vi "HEWH RLT Error Checker.vi"(0 "A Data Array":string[][](array[string]), 1 "Disable Station 1":T1, 2 "Disable Station 2":T1, 5 "B Data Array":string[][](array[string]), 7 "C Data Array":string[][](array[string]), 9 "D Data Array":string[][](array[string]), 11 "Error In":errorcluster, 12 "Disable Station 3":T1, 13 "Disable Station 4":T1) -> (4 "Alarm A":bool, 6 "Alarm B":bool, 8 "Alarm C":bool, 10 "Alarm D":bool, 15 "Error Out":errorcluster)   [LabVIEW 2016]
uses:
  Type Definitions/HEWH RLT Station Disable.ctl
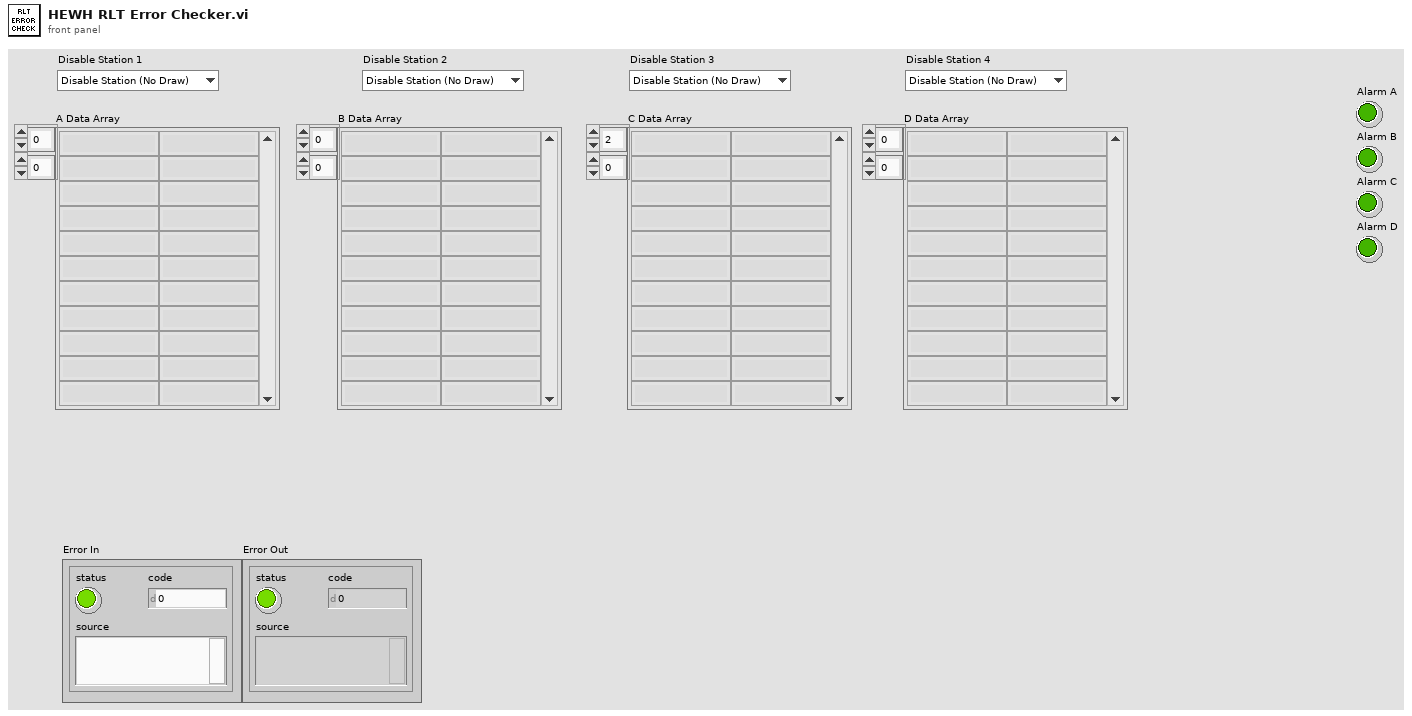
[diagram p1: front panel]
types:
  T1 = typedef "HEWH RLT Station Disable.ctl" = enum16{"Disable Station (No Draw)", "Enable Station"}
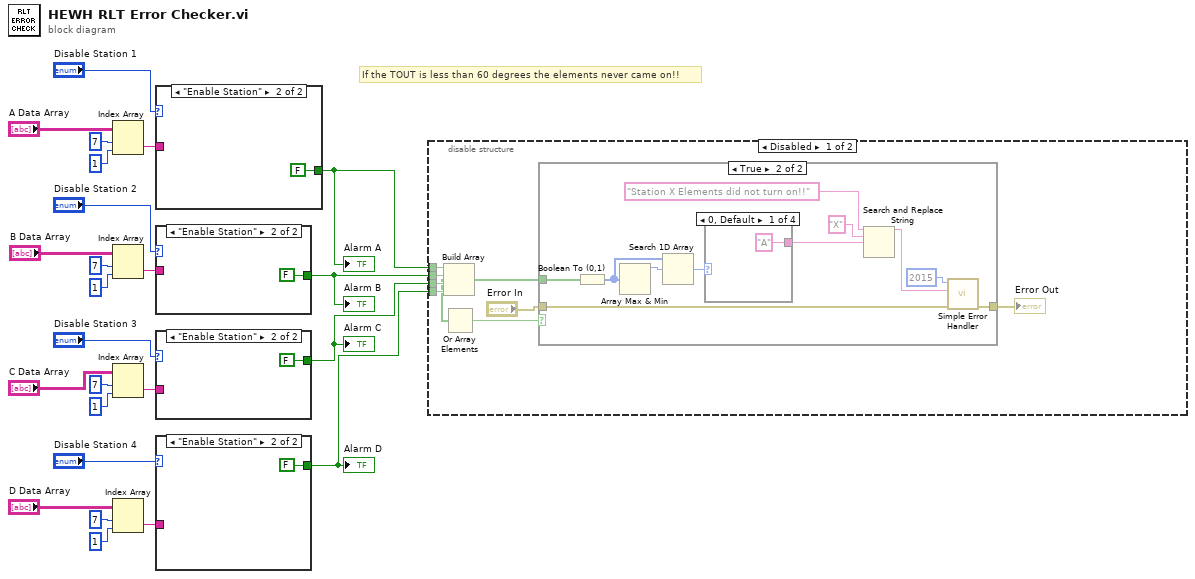
[diagram p0: block diagram]
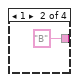
[diagram p3: hidden frame]
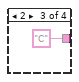
[diagram p4: hidden frame]
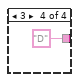
[diagram p5: hidden frame]
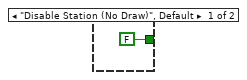
[diagram p7: hidden frame]
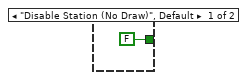
[diagram p8: hidden frame]
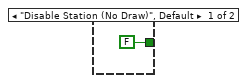
[diagram p9: hidden frame]
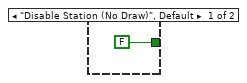
[diagram p10: hidden frame]
diagram:
  # "If the TOUT is less than 60 degrees the elements never came on!!"
  n1 = Index Array(array="A Data Array", index (row)=7 ("disabled index (row)"), index (col)=1 ("disabled index (col)")) -> (element=w11:string)
  n2 = Index Array(array="B Data Array", index (row)=7 ("disabled index (row)"), index (col)=1 ("disabled index (col)")) -> (element=w8:string)
  n3 = Index Array(array="C Data Array", index (row)=7 ("disabled index (row)"), index (col)=1 ("disabled index (col)")) -> (element=w9:string)
  n4 = Index Array(array="D Data Array", index (row)=7 ("disabled index (row)"), index (col)=1 ("disabled index (col)")) -> (element=w10:string)
  n5 = case shown="\"Enable Station\"" "Disable Station 1" {
    tunnel: w11 -> [_ _]
    tunnel: [FALSE FALSE] -> w4
    frame "Disable Station (No Draw)", Default {
    }
    frame "Enable Station" {
    }
  }
  "Alarm A" <- w4
  n6 = case shown="\"Enable Station\"" "Disable Station 2" {
    tunnel: w8 -> [_ _]
    tunnel: [FALSE FALSE] -> w3
    frame "Disable Station (No Draw)", Default {
    }
    frame "Enable Station" {
    }
  }
  "Alarm B" <- w3
  n7 = case shown="\"Enable Station\"" "Disable Station 3" {
    tunnel: w9 -> [_ _]
    tunnel: [FALSE FALSE] -> w2
    frame "Disable Station (No Draw)", Default {
    }
    frame "Enable Station" {
    }
  }
  "Alarm C" <- w2
  n8 = case shown="\"Enable Station\"" "Disable Station 4" {
    tunnel: w10 -> [_ _]
    tunnel: [FALSE FALSE] -> w1
    frame "Disable Station (No Draw)", Default {
    }
    frame "Enable Station" {
    }
  }
  "Alarm D" <- w1
  n9 = disable-structure shown="Disabled" {
    disable-tunnel: w4 -> [w40 _]
    disable-tunnel: w3 -> [w39 _]
    disable-tunnel: w2 -> [w38 _]
    disable-tunnel: w1 -> [w37 _]
    frame Disabled {
      n10 = Build Array(w40, w39, w38, w37) -> (w33:bool[])
      n11 = Or Array Elements(Boolean array=w33) -> (logical OR=w36:bool)
      n12 = case shown="True" w36 {
        tunnel: "Error In" -> [w41 w52]
        tunnel: [w41 w51] -> w34
        tunnel: w33 -> [_ w43]
        frame False {
        }
        frame True {
          n13 = Boolean To (0,1)(Boolean=w43) -> (0, 1=w45:i16[])
          n14 = Array Max & Min(array=w45) -> (max value=w44:i16)  [unwired: 3 out]
          n15 = Search 1D Array(1D array=w45, element=w44) -> (index of element=w46:i32)  [unwired: 1 in]
          n16 = case shown="0, Default" w46 {
            tunnel: ["A" ("search string") "B" ("search string") "C" ("search string") "D" ("search string")] -> w47
            frame 0, Default {
            }
            frame 1 {
            }
            frame 2 {
            }
            frame 3 {
            }
          }
          n17 = Search and Replace String(input string="Station X Elements did not turn on!!", search string="X", replace string=w47) -> (result string=w42:string)  [unwired: 5 in, 3 out]
          n18 = call <vilib>:"Simple Error Handler.vi"("error code (no error:0)"=2015, "error source (\" \")"=w42, "error in (no error)"=w52) -> ("error out"=w51:errorcluster)  [unwired: 2 in, 4 out]
        }
      }
      "Error Out" <- w34
    }
    frame Enabled {
    }
  }
